vi "Trial - Create New.vi"(8 "Error IN":errorcluster, 11 "Existing Recipe Names":string[](array[string])) -> (0 "Error OUT":errorcluster, 1 "Cancel OUT":bool, 3 "Enter New Recipe File Name OUT":string)   [LabVIEW 2018]
panel:
  out "Total Characters":dbl
  in  "Enter New Trial Config File Name":string
  in  "Cancel":bool
  in  "Next":bool
  # "New Trial File Name"
  # ".dat"
  # "*Note - File Name limited to 40 characters"
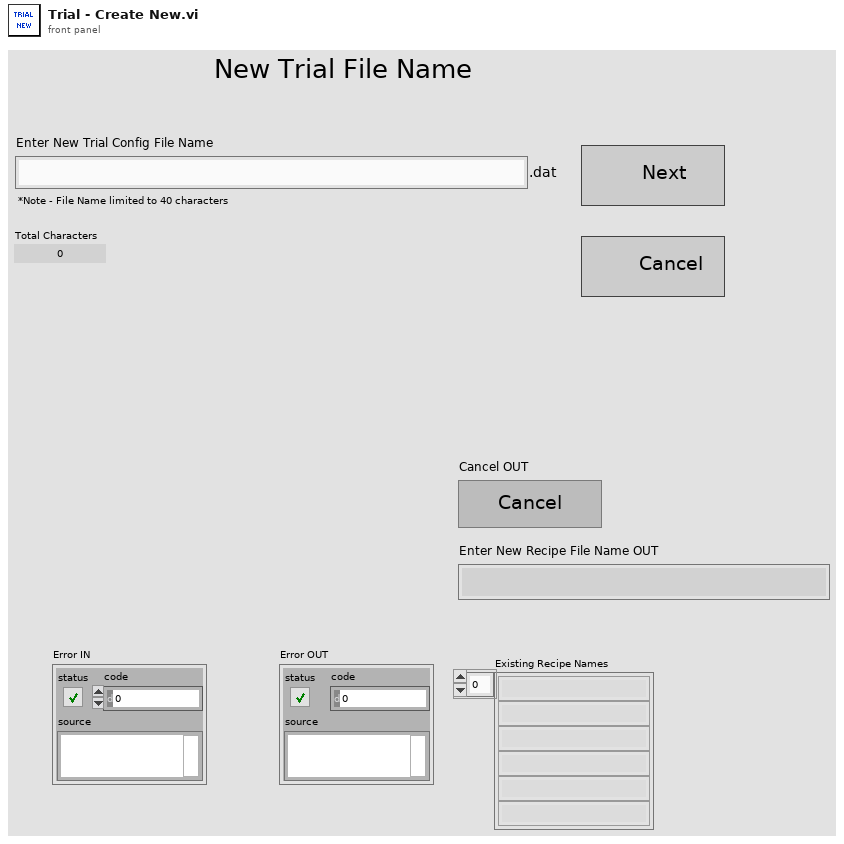
[diagram p1: front panel]
types:
  T1 = enum8{"Enabled", "Disabled", "Disabled and Grayed Out"}
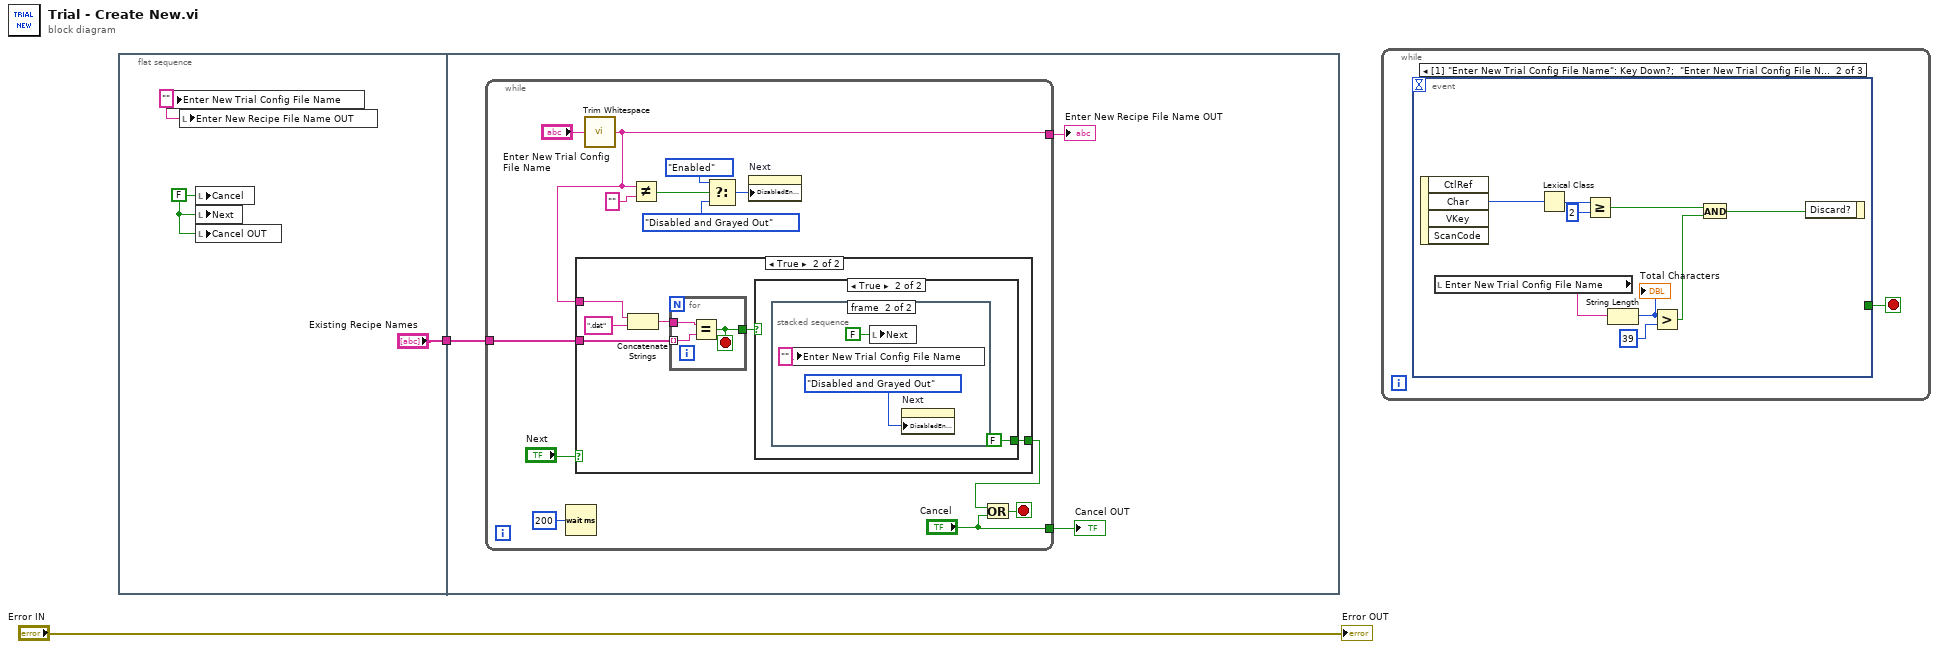
[diagram p0: block diagram]
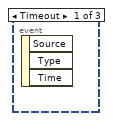
[diagram p2: hidden frame]
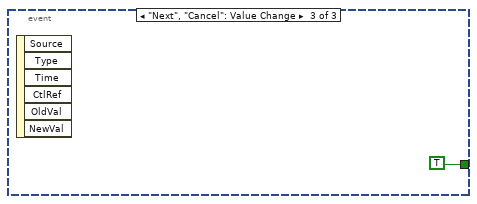
[diagram p3: hidden frame]
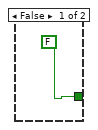
[diagram p4: hidden frame]
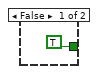
[diagram p5: hidden frame]
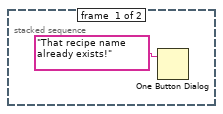
[diagram p6: hidden frame]
diagram:
  n1 = flat-sequence {
    tunnel: ["Existing Recipe Names"] -> w1
    tunnel: w1 -> [w7]
    frame #0 {
      w4 = FALSE ("Cancel")
      w5 = "" ("Enter New Recipe File Name")
      n2 = local write "Enter New Trial Config File Name"(w5) -> ()
      n3 = local write "Enter New Recipe File Name OUT"(w5) -> ()
      n4 = local write "Cancel"(w4) -> ()
      n5 = local write "Next"(w4) -> ()
      n6 = local write "Cancel OUT"(w4) -> ()
    }
    frame #1 {
      n7 = while {
        tunnel: [w9] -> w6
        tunnel: ["Cancel"] -> w8
        tunnel: w7 -> [w12]
        stop <- w21 stop-if-true
        n8 = Wait (ms)(milliseconds to wait=u32 200) -> ()  [unwired: 1 out]
        n9 = call <vilib>:"Trim Whitespace.vi"("string"="Enter New Trial Config File Name") -> ("trimmed string"=w9:string)  [unwired: 1 in]
        n10 = case shown="True" "Next" {
          tunnel: w9 -> [_ w25]
          tunnel: w12 -> [_ w28]
          tunnel: [FALSE w26] -> w11
          frame False {
          }
          frame True {
            n11 = Concatenate Strings(w25, ".dat" ("string")) -> (w24:string)
            n12 = for {
              tunnel: w28 -> [w36] mode=indexing
              tunnel: w24 -> [w37]
              tunnel: [w35] -> w27
              stop <- w35 stop-if-true
              n13 = Equal?(x=w37, y=w36) -> (x = y?=w35:bool)
            }
            n14 = case shown="True" w27 {
              tunnel: [TRUE FALSE] -> w26
              frame False {
              }
              frame True {
                n15 = stacked-sequence {
                  frame #0 {
                    n16 = One Button Dialog(message="That recipe name already exists!") -> ()  [unwired: 1 in, 1 out]
                  }
                  frame #1 {
                    n17 = local write "Enter New Trial Config File Name"("" ("Enter New Recipe File Name")) -> ()
                    n18 = local write "Next"(FALSE ("Next")) -> ()
                    n19 = property on="Next" class="Bool (strict)"("DisabledEnum"=T1."Disabled and Grayed Out" ("Disabled")) -> ()  [unwired: 2 in, 2 out]
                  }
                }
              }
            }
          }
        }
        n20 = Not Equal?(x=w9, y="") -> (x != y?=w18:bool)
        n21 = Select(t=T1."Enabled" ("Disabled"), s=w18, f=T1."Disabled and Grayed Out" ("Disabled")) -> (s? t:f=w15:T1)
        n22 = property on="Next" class="Bool (strict)"("DisabledEnum"=w15) -> ()  [unwired: 2 in, 2 out]
        n23 = Or(x=w11, y="Cancel") -> (x .or. y?=w21:bool)
      }
      "Enter New Recipe File Name OUT" <- w6
      "Cancel OUT" <- w8
    }
  }
  n24 = while {
    stop <- w38 stop-if-true
    n25 = event shown="[1] \"Enter New Trial Config File Name\": Key Down?;  \"Enter New Trial Config File Name\": Key Repeat?" {
      selector: _ -> [_ _ _]
      dyn-events: _ -> [_ _ _]
      timeout: _ -> [_ _ _]
      tunnel: [_ _ TRUE] -> w38
      event Timeout {
        n26 = event-data() -> ()  [unwired: 1 in, 3 out]
      }
      event "Enter New Trial Config File Name": Key Down?; "Enter New Trial Config File Name": event type 3.0.x8000000b {
        n27 = event-data() -> ("Char"=w47:i16)  [unwired: 1 in, 3 out]
        n28 = local read "Enter New Trial Config File Name"() -> (w43:string)
        n29 = Lexical Class(1:w47) -> (0:w46:i16)
        n30 = Greater Or Equal?(x=w46, y=i16 2) -> (x >= y?=w44:bool)
        n31 = String Length(string=w43) -> (length=w42:i32)
        "Total Characters" <- w42
        n32 = Greater?(x=w42, y=39) -> (0:w40:bool)
        n33 = And(x=w44, y=w40) -> (x .and. y?=w39:bool)
        n34 = event-data("Discard?"=w39) -> ()  [unwired: 1 in, 1 out]
      }
      event "Next", "Cancel": Value Change {
        n35 = event-data() -> ()  [unwired: 1 in, 6 out]
      }
    }
  }
  "Error OUT" <- "Error IN"
